vi "benchmarks_fileSHA1.vi"() -> ()   [LabVIEW 2013]
uses:
  SHA-1/SHA-1.lvclass
  <vilib>/Analysis/baseanly.llb/Mean (DBL).vi
  SHA-1/Enqueue File.vi
  SHA-1/pad.vi
  <vilib>/Analysis/NI_AALBase.lvlib
  SHA-1/SHA-1.lvlib
  <vilib>/MediaMongrels Ltd/WebSockets/WebSockets/WebSocket/WebSocket.lvclass
panel:
  out "equal hashes":bool
  out "% gain":dbl
  out "LVOS":dbl
  out "NI Forums":dbl
  in  "filepath":path
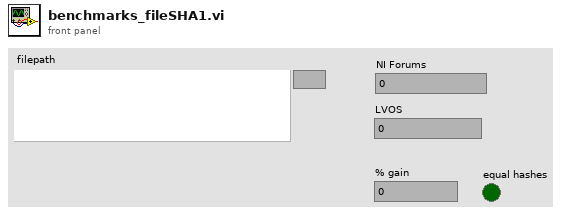
[diagram p1: front panel]
types:
  T1 = enum16{"open", "replace", "create", "open or create", "replace or create", "replace or create with confirmation"}
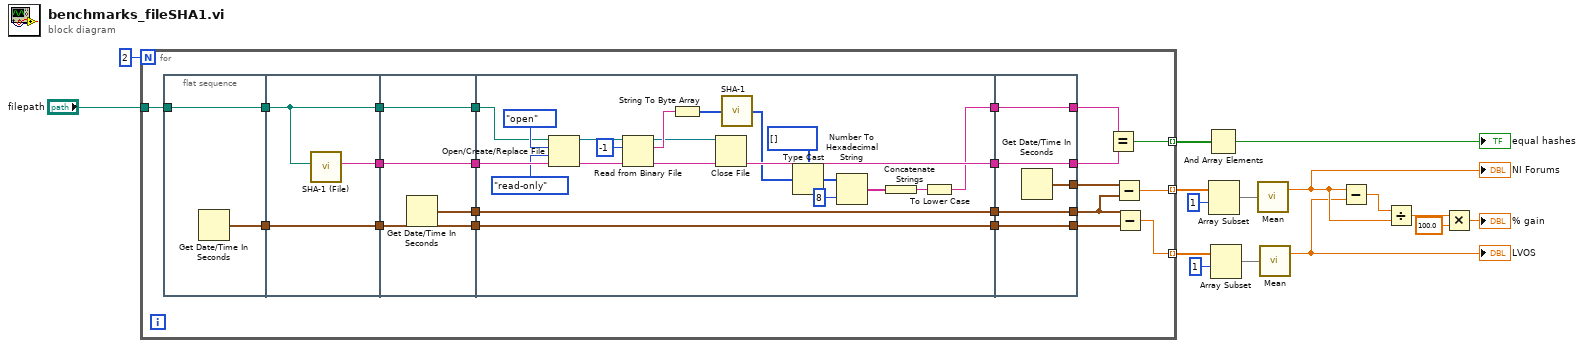
[diagram p0: block diagram]
diagram:
  n1 = for {
    N: 2 -> [_]
    tunnel: "filepath" -> [w25]
    tunnel: [w19] -> w15 mode=indexing
    tunnel: [w18] -> w8 mode=indexing
    tunnel: [w17] -> w7 mode=indexing
    n2 = flat-sequence {
      tunnel: w25 -> [w40]
      tunnel: [w40] -> w38
      tunnel: [w39] -> w37
      tunnel: [w42] -> w36
      tunnel: w38 -> [w42]
      tunnel: w37 -> [w43]
      tunnel: [w43] -> w35
      tunnel: [w41] -> w34
      tunnel: w36 -> [w47]
      tunnel: [w47] -> w33
      tunnel: [w46] -> w32
      tunnel: [w45] -> w31
      tunnel: w35 -> [w45]
      tunnel: [w44] -> w30
      tunnel: w34 -> [w44]
      tunnel: w33 -> [w55]
      tunnel: [w67] -> w29
      tunnel: w32 -> [w67]
      tunnel: [w66] -> w28
      tunnel: w31 -> [w66]
      tunnel: [w48] -> w27
      tunnel: [w65] -> w26
      tunnel: w30 -> [w65]
      tunnel: [w72] -> w23
      tunnel: w29 -> [w72]
      tunnel: [w71] -> w22
      tunnel: w28 -> [w71]
      tunnel: [w70] -> w24
      tunnel: [w69] -> w21
      tunnel: w27 -> [w69]
      tunnel: [w68] -> w20
      tunnel: w26 -> [w68]
      frame #0 {
        n3 = Get Date/Time In Seconds() -> (seconds since 1Jan1904=w39:timestamp)
      }
      frame #1 {
        n4 = call "SHA-1 (File).vi"("filepath"=w42) -> ("SHA-1 hash"=w41:string)  [unwired: 10 in]
      }
      frame #2 {
        n5 = Get Date/Time In Seconds() -> (seconds since 1Jan1904=w46:timestamp)
      }
      frame #3 {
        n6 = Open/Create/Replace File(file path (use dialog)=w55, operation (0:open)=T1."open", access (0:read/write)=enum16{"read/write", "read-only", "write-only"}."read-only") -> (refnum out=w58:refnum<file>, error out=w59:errorcluster)  [unwired: 3 in, 1 out]
        n7 = Read from Binary File(8:w59, 10:-1 ("count (1)"), 11:w58) -> (0:w62:errorcluster, 2:w63:string, 3:w61:refnum<file>)  [unwired: 3 in, 1 out]
        n8 = String To Byte Array(string=w63) -> (unsigned byte array=w64:u8[])
        n9 = Close File(refnum=w61, error in=w62) -> ()  [unwired: 2 out]
        n10 = call <vilib>:"SHA-1.vi"("Data"=w64) -> ("message-digest"=w49:u8[])
        n11 = Type Cast(type=u32[] [] ("U32"), x=w49) -> (*(type *) &x=w52:u32[])
        n12 = Number To Hexadecimal String(1:i16 8 ("width (-)"), 2:w52) -> (0:w51:string[])
        n13 = Concatenate Strings(w51) -> (w50:string)
        n14 = To Lower Case(string=w50) -> (all lower case string=w48:string)
      }
      frame #4 {
        n15 = Get Date/Time In Seconds() -> (seconds since 1Jan1904=w70:timestamp)
      }
    }
    n16 = Equal?(x=w21, y=w20) -> (x = y?=w19:bool)
    n17 = Subtract(x=w24, y=w23) -> (x-y=w18:dbl)
    n18 = Subtract(x=w23, y=w22) -> (x-y=w17:dbl)
  }
  n19 = And Array Elements(Boolean array=w15) -> (logical AND=→"equal hashes":bool)
  n20 = Array Subset(array=w8, index=1) -> (w11:dbl[])  [unwired: 1 in]
  n21 = Array Subset(array=w7, index=1) -> (w10:dbl[])  [unwired: 1 in]
  n22 = call-poly <vilib>:"Mean.vi"("X"=w11) -> ("mean"=w3:dbl)  [unwired: 1 out]
  "NI Forums" <- w3
  n23 = call-poly <vilib>:"Mean.vi"("X"=w10) -> ("mean"=w2:dbl)  [unwired: 1 out]
  "LVOS" <- w2
  n24 = Subtract(x=w3, y=w2) -> (x-y=w6:dbl)
  n25 = Divide(x=w6, y=w3) -> (x/y=w4:dbl)
  n26 = Multiply(x=w4, y=100.0) -> (x*y=→"% gain":dbl)
